vi "SERIAL_GlobalYawOffset.vi"(10 "InputYawOffset":dbl format="%#_13g", 11 "Set":bool=TRUE) -> (3 "OutputYawOffset":dbl format="%#_13g")   [LabVIEW 2014, in "navX-MXP IMU.lvlib"]
uses:
  navX-MXP IMU.lvlib
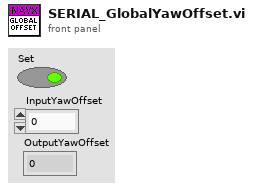
[diagram p1: front panel]
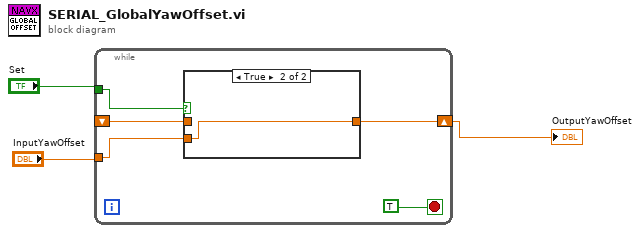
[diagram p0: block diagram]
diagram:
  n1 = while {
    shift-right: [w5] -> w1
    shift-left: _ -> [w4]
    tunnel: "InputYawOffset" -> [w6]
    tunnel: "Set" -> [w7]
    stop <- TRUE stop-if-true
    n2 = case shown="True" w7 {
      tunnel: w6 -> [_ w10]
      tunnel: [w9 w10] -> w5
      tunnel: w4 -> [w9 _]
      frame False {
      }
      frame True {
      }
    }
  }
  "OutputYawOffset" <- w1
